vi "Get Formated String.vi"(8 "error in (no error)":errorcluster, 11 "Words to Numbers Converter in":refnum<class "Words to Numbers Converter.lvclass">) -> (0 "error out":errorcluster, 2 "String":string, 3 "Words to Numbers Converter out":refnum<class "Words to Numbers Converter.lvclass">)   [LabVIEW 2020, in "Words to Numbers Converter.lvclass"]
uses:
  Words to Numbers Converter.lvclass
  Words to Numbers Converter.lvclass/Words to Numbers Converter.ctl
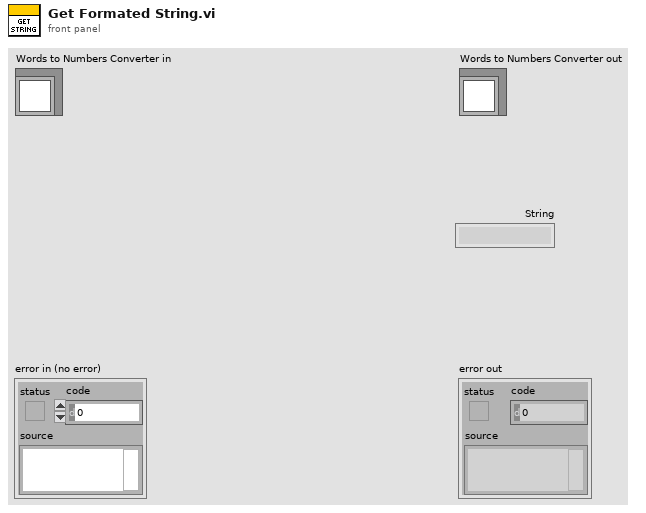
[diagram p1: front panel]
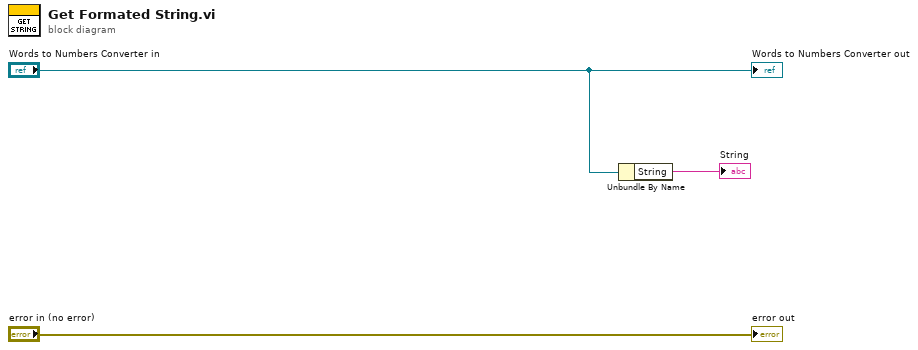
[diagram p0: block diagram]
diagram:
  n1 = Unbundle By Name("Words to Numbers Converter in") -> ("String"=→"String":string)
  "error out" <- "error in (no error)"
  "Words to Numbers Converter out" <- "Words to Numbers Converter in"
